vi "Pre Launch Init.vi"(11 "Nested in":refnum<class "UI Actor.lvclass">) -> (0 "error out":errorcluster, 3 "Nested out":refnum<class "UI Actor.lvclass">)   [LabVIEW 2019, in "UI Actor.lvlib" / "UI Actor.lvclass"]
doc: "(<B>Filename</B>: Actor Framework.lvlib:Actor.lvclass:Pre Launch Init.vi)\n\nDefines behavior that occurs after the Launch Nested Actor method is invoked but before the actor's Actor Core method begins running.\n\nBy default, this method does nothing. A descendant class may override it to define behavior."
uses:
  UI Actor.lvclass
  C:/Program Files/National Instruments/LabVIEW 2019/vi.lib/ActorFramework/Actor/Actor.lvclass
  UI Actor.lvclass/UI Actor.ctl
  <vilib>/ActorFramework/Actor/Actor.lvclass/Actor.ctl
  <vilib>/ActorFramework/Message Enqueuer/Message Enqueuer.lvclass/Message Enqueuer.ctl
  <vilib>/ActorFramework/Message Enqueuer/Init from Existing Queue.vi
  <vilib>/ActorFramework/Message Enqueuer/Enqueue.vi
  UI Actor Messages/Init Msg/Init Msg.lvclass
  C:/Program Files/National Instruments/LabVIEW 2019/vi.lib/ActorFramework/Message/Message.lvclass
  <vilib>/ActorFramework/Message Priority Queue/Priority Enqueue.vi
  <vilib>/ActorFramework/Message Enqueuer/Message Enqueuer.lvclass
  <vilib>/ActorFramework/Actor/Actor.lvclass
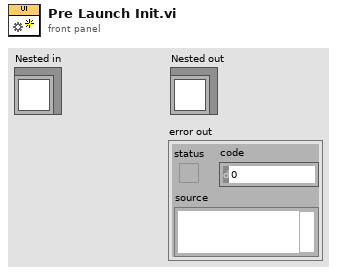
[diagram p1: front panel]
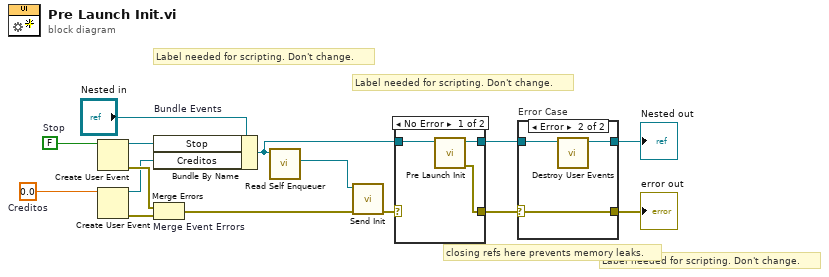
[diagram p0: block diagram]
diagram:
  w3 = 0.0  # Creditos
  w14 = FALSE  # Stop
  # "Label needed for scripting. Don't change."
  # "Label needed for scripting. Don't change."
  # "Label needed for scripting. Don't change."
  # "closing refs here prevents memory leaks."
  n1 = Create User Event(user event datatype=w14) -> (user event=w11:refnum<user-event>, error out=w13:errorcluster)  [unwired: 1 in]
  n2 = Create User Event(user event datatype=w3) -> (user event=w2:refnum<user-event>, error out=w1:errorcluster)  [unwired: 1 in]
  n3 = Bundle By Name "Bundle Events"(cluster="Nested in", "Stop"=w11, "Creditos"=w2) -> (w7:refnum<class "UI Actor.lvclass">)
  n4 = Merge Errors "Merge Event Errors"(w13, w1) -> (w6:errorcluster)
  n5 = call <vilib>:"Read Self Enqueuer.vi"("Actor"=w7) -> ("Self Enqueuer"=w4:refnum<class "Message Enqueuer.lvclass">)  [unwired: 10 in]
  n6 = call "Send Init.vi"("error in (no error)"=w6, "Message Enqueuer"=w4) -> ("error out"=w5:errorcluster)  [unwired: 8 in, 1 out]
  n7 = case shown="No Error" w5 {
    selector: w5 -> [_ w20]
    tunnel: [w18 w19] -> w9
    tunnel: w7 -> [w17 w19]
    tunnel: [w16 w20] -> w8
    frame No Error {
      n8 = call-parent "Pre Launch Init.vi"("Actor in"=w17) -> ("error out"=w16:errorcluster, "Actor out"=w18:refnum<class "UI Actor.lvclass">)  [unwired: 9 in]
    }
    frame Error {
    }
  }
  n9 = case "Error Case" shown="Error" w8 {
    selector: w8 -> [w21 w25]
    tunnel: w9 -> [w22 w24]
    tunnel: [w22 w23] -> w12
    tunnel: [w21 w25] -> w10
    frame No Error {
    }
    frame Error {
      n10 = call "Destroy User Events.vi"("UI Template in"=w24) -> ("UI Template out"=w23:refnum<class "UI Actor.lvclass">)  [unwired: 10 in]
    }
  }
  "error out" <- w10
  "Nested out" <- w12
